vi "ASDA-A2_Read Register Data.vi"(8 "error in":errorcluster, 10 "Read Register Data":T1 {"Address" format="%.0x"}, 11 "Buffer Data In":T2) -> (0 "error out":errorcluster, 2 "Data":u16[](array[numeric]), 3 "Buffer Data Out":T2)   [LabVIEW 2016]
uses:
  Data Def/ASDA-A2_Buffer Data.ctl
  Data Def/ASDA-A2_Read Register Data.ctl
  <vilib>/Modbus/master/Modbus Master.lvclass
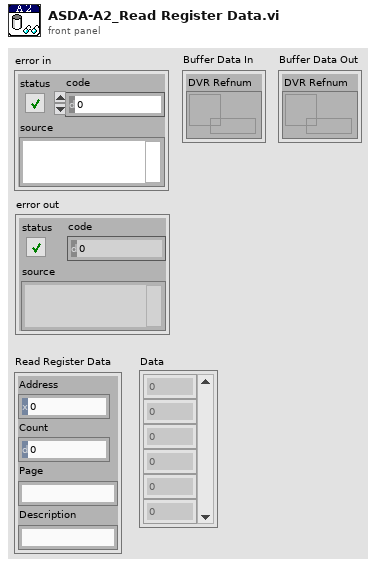
[diagram p1: front panel]
types:
  T1 = typedef "ASDA-A2_Read Register Data.ctl" = cluster{"Address":u16, "Count":u16, "Page":string, "Description":string}
  T2 = typedef "ASDA-A2_Buffer Data.ctl" = cluster{"DVR Refnum":refnum<data-value>}
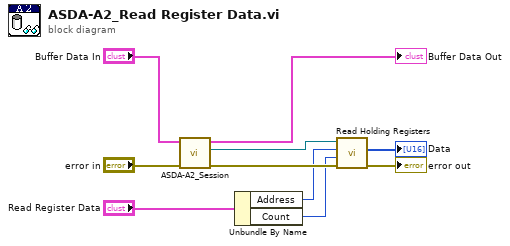
[diagram p0: block diagram]
diagram:
  n1 = call "ASDA-A2_Session.vi"("error in"="error in", "Buffer Data In"="Buffer Data In") -> ("error out"=w8:errorcluster, "Session Out"=w7:refnum<class "Modbus Master.lvclass">, "Buffer Data Out"=→"Buffer Data Out":T2)  [unwired: 7 in]
  n2 = Unbundle By Name("Read Register Data") -> ("Address"=w3:u16, "Count"=w2:u16)
  n3 = call-dynamic "Read Holding Registers.vi"("error in (no error)"=w8, "number of holding registers"=w2, "starting address"=w3, "Modbus master in"=w7) -> ("error out"=→"error out":errorcluster, "register values"=→"Data":u16[])  [unwired: 5 in, 1 out]
